vi "Read Broker Path.vi"(8 "error in":errorcluster, 11 "System in":refnum<class "System.lvclass">) -> (0 "error out":errorcluster, 2 "Broker Path":path, 3 "System out":refnum<class "System.lvclass">)   [LabVIEW 2014, in "System.lvclass"]
uses:
  System.lvclass
  System.lvclass/System.ctl
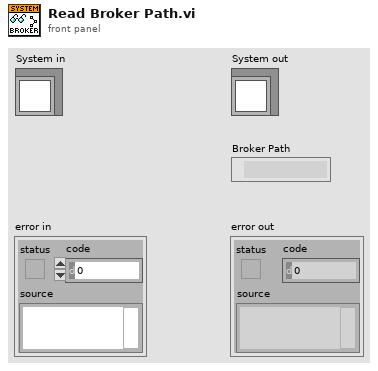
[diagram p1: front panel]
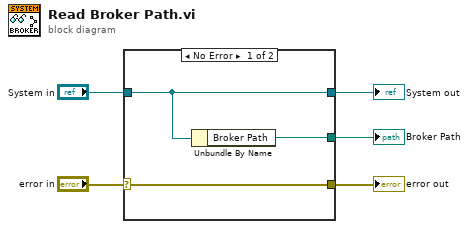
[diagram p0: block diagram]
diagram:
  n1 = case shown="No Error" "error in" {
    selector: "error in" -> [w8 w9]
    tunnel: [w8 w9] -> w4
    tunnel: [w7 w10] -> w2
    tunnel: "System in" -> [w7 w10]
    tunnel: [w6 _] -> w1
    frame No Error {
      n2 = Unbundle By Name(w7) -> ("Broker Path"=w6:path)
    }
    frame Error {
    }
  }
  "error out" <- w4
  "System out" <- w2
  "Broker Path" <- w1
